vi "Card_detection.vi"(8 "error in (no error)":errorcluster, 10 "Card":bool, 11 "Card_detection in":refnum<class "Card_detection.lvclass">) -> (0 "error out":errorcluster, 3 "State out":refnum<class "State Actor.lvclass">)   [LabVIEW 2025, in "User_Console-ATM.lvlib" / "Card_detection.lvclass"]
uses:
  Card_detection.lvclass
  <vilib>/ni/Actors/State Actor/State Actor/State Actor.lvclass
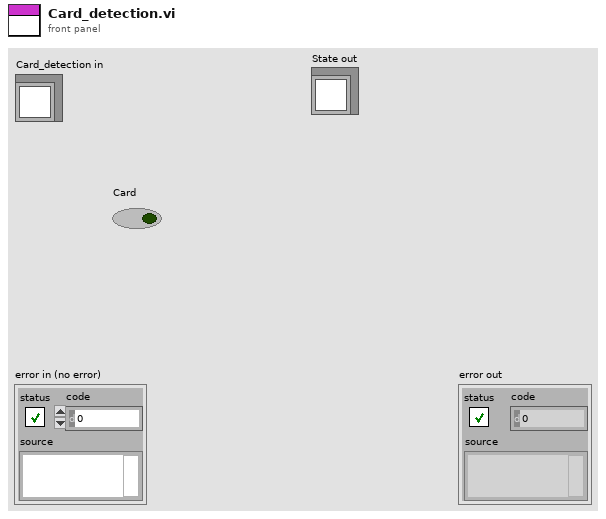
[diagram p1: front panel]
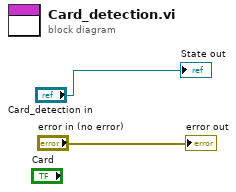
[diagram p0: block diagram]
diagram:
  "error out" <- "error in (no error)"
  "State out" <- "Card_detection in"
